vi "GetComparison.vi"(8 "error in":errorcluster, 11 "BooleanMeasureLimit in":refnum<class "BooleanMeasureLimit.lvclass">) -> (0 "error out":errorcluster, 2 "Comparison":bool, 3 "BooleanMeasureLimit out":refnum<class "BooleanMeasureLimit.lvclass">)   [LabVIEW 2021, in "ProligentXMLGenerator.lvlib" / "BooleanMeasureLimit.lvclass"]
doc: "Boolean Measure Limit Comparison"
uses:
  BooleanMeasureLimit.lvclass
  BooleanMeasureLimit.lvclass/BooleanMeasureLimit.ctl
  Base/Boolean/Boolean.lvclass
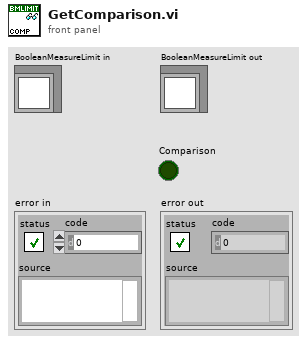
[diagram p1: front panel]
types:
  T1 = typedef "ProligentXMLGenerator.lvlib/BooleanMeasureLimit.lvclass/Data.ctl" = cluster{"Comparison":refnum<class "Boolean.lvclass">}
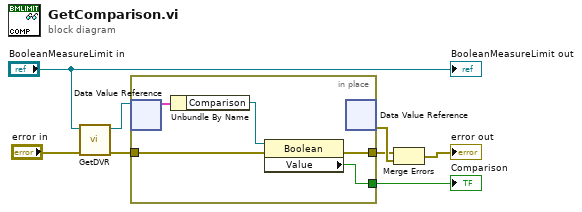
[diagram p0: block diagram]
diagram:
  n1 = call "GetDVR.vi"("error in"="error in", "BooleanMeasureLimit"="BooleanMeasureLimit in") -> ("error out"=w4:errorcluster, "DVRReference"=w3:refnum<data-value>)  [unwired: 8 in]
  n2 = in-place "In Place Element Structure" {
    in-place-border: [w9] -> w1
    in-place-border: w4 -> [w11]
    in-place-border: [w10] -> w5
    n3 = in-place-dvr #1(w3) -> (w13:T1)  [unwired: 1 out]
    n4 = Unbundle By Name(w13) -> ("Comparison"=w12:refnum<class "Boolean.lvclass">)
    n5 = property class="Boolean"(reference=w12, error in=w11) -> (error out=w10:errorcluster, "Value"=w9:bool)  [unwired: 1 out]
    n6 = in-place-dvr #1() -> (w6:errorcluster)  [unwired: 1 in, 1 out]
  }
  "Comparison" <- w1
  n7 = Merge Errors(w5, w6) -> (→"error out":errorcluster)
  "BooleanMeasureLimit out" <- "BooleanMeasureLimit in"
